vi "Build Robot.vi"(8 "error in":errorcluster, 10 "Robotic Parts":T1[](array[typedef])) -> (0 "error out":errorcluster, 1 "Scene Out":refnum<vi>, 2 "Joint Array":T4[](array[typedef]))   [LabVIEW 2015]
doc: "This VI generates the3D picture of the robot in the simulation"
uses:
  <vilib>/robotics/Kinematics/Plotting/Joint Control.ctl
  <vilib>/robotics/Kinematics/Plotting/Joint Type.ctl
  Controls/Robotic Parts.ctl
  <vilib>/robotics/Kinematics/Plotting/Element Type.ctl
  <vilib>/picture/3D Picture Control/Object/Create Object (name).vi
  <vilib>/picture/3D Picture Control/NI_3D Picture Control.lvlib
  <vilib>/robotics/Kinematics/Plotting/NI_Robotics_3DKinematics.lvlib
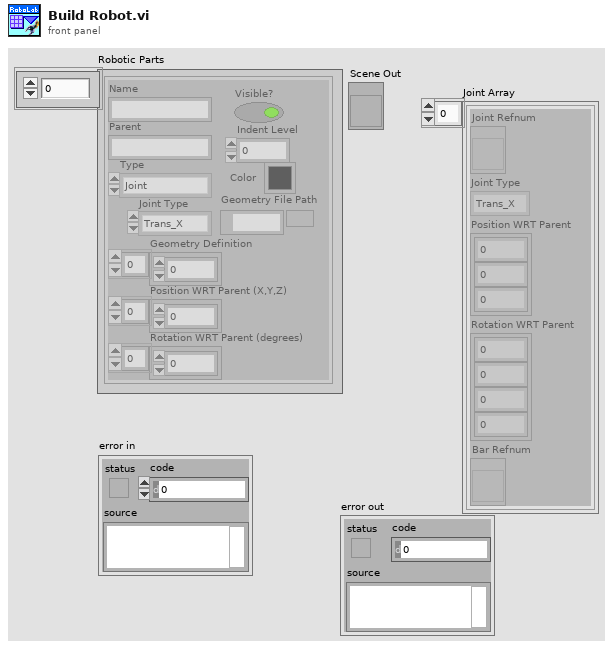
[diagram p1: front panel]
types:
  T1 = typedef "Robotic Parts.ctl" = cluster{"Name":string, "Parent":string, "Type":T2, "Visible?":bool, "Geometry Definition":dbl[], "Position WRT Parent (X,Y,Z)":dbl[], "Rotation WRT Parent (degrees)":dbl[], "Joint Type":T3, "Geometry File Path":path, "Indent Level":i32, "Color":u32}
  T2 = typedef "NI_Robotics_3DKinematics.lvlib/Element Type.ctl" = enum16{"Joint", "Box", "Cylinder", "Cone", "Sphere", "ASE File", "VRML File", "STL File", "Space"}
  T3 = typedef "NI_Robotics_3DKinematics.lvlib/Joint Type.ctl" = enum16{"Trans_X", "Trans_Y", "Trans_Z", "Rot_X", "Rot_Y", "Rot_Z", "None"}
  T4 = typedef "NI_Robotics_3DKinematics.lvlib/Joint Control.ctl" = cluster{"Joint Refnum":refnum<vi>, "Joint Type":T3, "Position WRT Parent":dbl[], "Rotation WRT Parent":dbl[], "Bar Refnum":refnum<vi>}
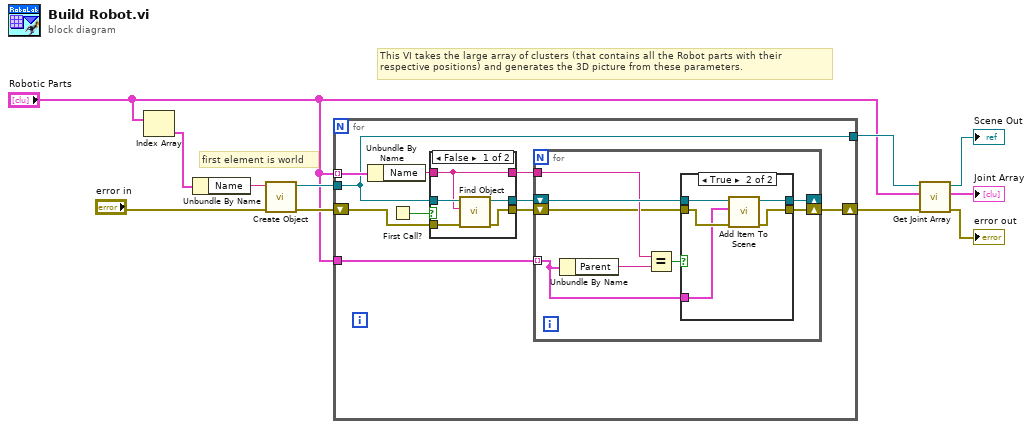
[diagram p0: block diagram]
diagram:
  # "This VI takes the large array of clusters (that contains all the Robot parts with their\nrespective positions) and generates the 3D picture from these parameters."
  # "first element is world"
  n1 = Index Array(array="Robotic Parts") -> (element=w9:T1)  [unwired: 1 in]
  n2 = Unbundle By Name(w9) -> ("Name"=w8:string)
  n3 = call-poly <vilib>:"Create Object.vi"("error in (no error)"="error in", "Name"=w8) -> ("error out"=w11:errorcluster, "Scene:New Object"=w10:refnum<vi>)  [unwired: 8 in]
  n4 = for {
    tunnel: "Robotic Parts" -> [w21]
    tunnel: "Robotic Parts" -> [w20] mode=indexing
    shift-right: [w15] -> w5
    shift-left: w11 -> [w14]
    tunnel: [w12] -> w6
    tunnel: w10 -> [w12]
    n5 = Unbundle By Name(w20) -> ("Name"=w16:string)
    n6 = First Call?() -> (First Call?: T/F=w19:bool)
    n7 = case shown="False" w19 {
      tunnel: w12 -> [w26 w29]
      tunnel: [w25 w29] -> w18
      tunnel: [w24 w28] -> w17
      tunnel: w16 -> [w24 w28]
      tunnel: w14 -> [w23 w27]
      tunnel: [w22 w27] -> w13
      frame False {
        n8 = call <vilib>:"Find Object.vi"("error in (no error)"=w23, "Object Name"=w24, "Scene Refnum"=w26) -> ("error out"=w22:errorcluster, "Object Refnum"=w25:refnum<vi>)  [unwired: 7 out]
      }
      frame True {
      }
    }
    n9 = for {
      tunnel: w21 -> [w35] mode=indexing
      shift-right: [w30] -> _
      shift-left: w18 -> [w34]
      tunnel: w17 -> [w33]
      shift-right: [w32] -> w15
      shift-left: w13 -> [w31]
      n10 = Unbundle By Name(w35) -> ("Parent"=w37:string)
      n11 = Equal?(x=w33, y=w37) -> (x = y?=w36:bool)
      n12 = case shown="True" w36 {
        tunnel: w34 -> [w39 w44]
        tunnel: w35 -> [_ w40]
        tunnel: [w39 w43] -> w30
        tunnel: [w38 w42] -> w32
        tunnel: w31 -> [w38 w41]
        frame False {
        }
        frame True {
          n13 = call "Add Item To Scene.vi"("error in"=w41, "Tree Element"=w40, "Scene In"=w44) -> ("error out"=w42:errorcluster, "Scene Out"=w43:refnum<vi>)  [unwired: 7 in]
        }
      }
    }
  }
  n14 = call "Get Joint Array.vi"("error in"=w5, "Tree Elements"="Robotic Parts", "Scene In"=w6) -> ("error out"=→"error out":errorcluster, "Joint Array"=→"Joint Array":T4[], "Scene Out"=→"Scene Out":refnum<vi>)  [unwired: 6 in]
